vi "Exit with Code.vi"(8 "error in (no error)":errorcluster, 10 "Exit Code (0)":i32, 11 "CLI in":refnum<class "CLI.lvclass">) -> (0 "error out":errorcluster)   [LabVIEW 2017, in "CLI.lvclass"]
doc: "Ends the command line executable with the exit code provided.\n\nCall this when your application ends to ensure the caller see's that it has ended."
uses:
  CLI.lvclass
  CLI.lvclass/CLI.ctl
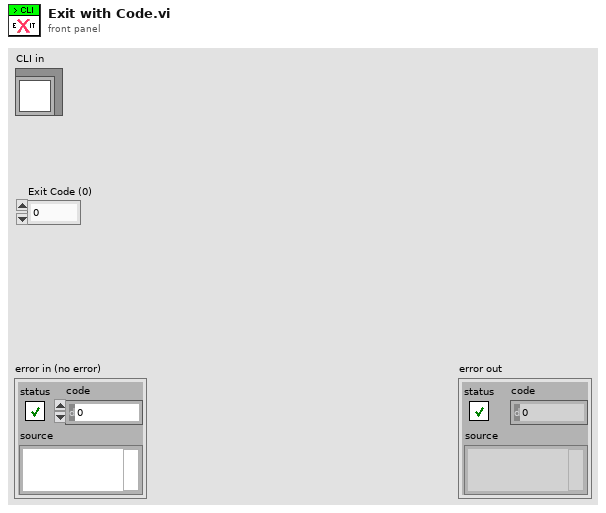
[diagram p1: front panel]
types:
  T1 = typedef "Events.ctl" = cluster{"STIN":refnum<user-event>, "SIGI":refnum<user-event>, "UnknownSignal":refnum<user-event>}
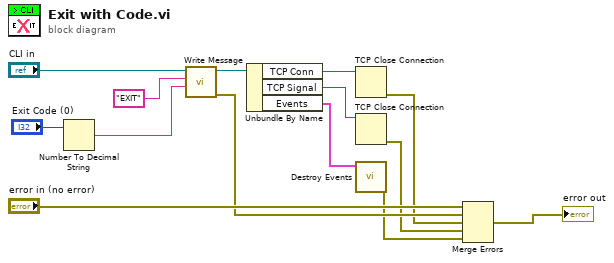
[diagram p0: block diagram]
diagram:
  n1 = Number To Decimal String(number="Exit Code (0)") -> (decimal integer string=w5:string)  [unwired: 1 in]
  n2 = call "Write Message.vi"("Message Contents"=w5, "Message Type"="EXIT", "CLI in"="CLI in") -> ("error out"=w7:errorcluster, "CLI out"=w10:refnum<class "CLI.lvclass">)  [unwired: 7 in]
  n3 = Unbundle By Name(w10) -> ("TCP Conn"=w9:refnum<k5>, "TCP Signal"=w4:refnum<k5>, "Events"=w2:T1)
  n4 = TCP Close Connection(connection ID=w9) -> (error out=w6:errorcluster)  [unwired: 2 in, 1 out]
  n5 = TCP Close Connection(connection ID=w4) -> (error out=w3:errorcluster)  [unwired: 2 in, 1 out]
  n6 = call "Destroy Events.vi"("Events"=w2) -> ("error out"=w1:errorcluster)  [unwired: 10 in]
  n7 = Merge Errors("error in (no error)", w7, w6, w3, w1) -> (→"error out":errorcluster)
